vi "Enqueue_data(SubVI).vi"(6 "Numeric":i32, 8 "error in (no error)":errorcluster, 9 "Errors":dbl[][](array[numeric]), 10 "PIDs":dbl[](array[numeric]), 11 "Queue in":refnum<queue>) -> (0 "error out":errorcluster, 3 "Queue out":refnum<queue>)   [LabVIEW 2017]
doc: "SubVI that enque data to queue.\nIt can only take one array in at a time, either PIDs or Errors.\nPIDs table is extended of information in which loop that table was obtained then its enqueued while Errors is divided into 3 subarrays that are enqueued to queue."
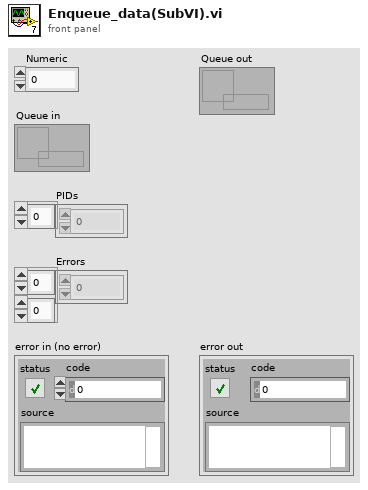
[diagram p1: front panel]
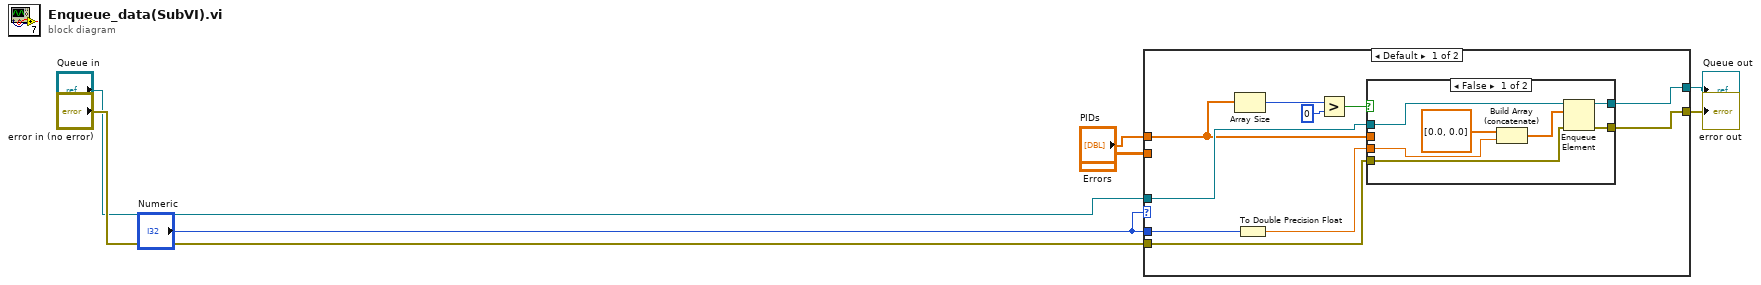
[diagram p0: block diagram]
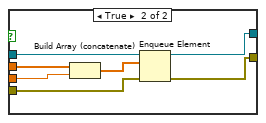
[diagram p2: hidden frame]
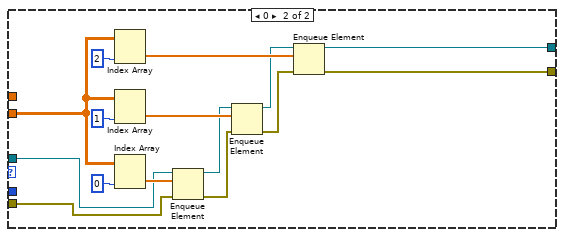
[diagram p3: hidden frame]
diagram:
  n1 = case shown="Default" "Numeric" {
    tunnel: "Errors" -> [_ w43]
    tunnel: [w12 w37] -> w2
    tunnel: "Numeric" -> [w17 _]
    tunnel: "Queue in" -> [w15 w36]
    tunnel: "error in (no error)" -> [w16 w35]
    tunnel: [w13 w32] -> w6
    tunnel: "PIDs" -> [w11 _]
    frame Default {
      n2 = Array Size(array=w11) -> (size(s)=w10:i32)
      n3 = To Double Precision Float(number=w17) -> (double precision float=w14:dbl)
      n4 = Greater?(x=w10, y=0) -> (0:w8:bool)
      n5 = case shown="False" w8 {
        tunnel: w16 -> [w22 w31]
        tunnel: w15 -> [w24 w30]
        tunnel: w14 -> [w19 w29]
        tunnel: [w21 w27] -> w13
        tunnel: [w23 w26] -> w12
        tunnel: w11 -> [_ w25]
        frame False {
          n6 = Build Array (concatenate)(dbl[] [0.0, 0.0], w19) -> (w18:dbl[])
          n7 = Enqueue Element(queue=w24, element=w18, error in (no error)=w22) -> (queue out=w23:refnum<queue>, error out=w21:errorcluster)  [unwired: 1 in, 1 out]
        }
        frame True {
          n8 = Build Array (concatenate)(w25, w29) -> (w28:dbl[])
          n9 = Enqueue Element(queue=w30, element=w28, error in (no error)=w31) -> (queue out=w26:refnum<queue>, error out=w27:errorcluster)  [unwired: 1 in, 1 out]
        }
      }
    }
    frame 0 {
      n10 = Index Array(array=w43, index (col)=2 ("disabled index (col)")) -> (element=w40:dbl[])  [unwired: 1 in]
      n11 = Index Array(array=w43, index (col)=1 ("disabled index (col)")) -> (element=w41:dbl[])  [unwired: 1 in]
      n12 = Index Array(array=w43, index (col)=0 ("disabled index (col)")) -> (element=w42:dbl[])  [unwired: 1 in]
      n13 = Enqueue Element(queue=w36, element=w42, error in (no error)=w35) -> (queue out=w38:refnum<queue>, error out=w34:errorcluster)  [unwired: 1 in, 1 out]
      n14 = Enqueue Element(queue=w38, element=w41, error in (no error)=w34) -> (queue out=w39:refnum<queue>, error out=w33:errorcluster)  [unwired: 1 in, 1 out]
      n15 = Enqueue Element(queue=w39, element=w40, error in (no error)=w33) -> (queue out=w37:refnum<queue>, error out=w32:errorcluster)  [unwired: 1 in, 1 out]
    }
  }
  "error out" <- w6
  "Queue out" <- w2
